vi "File_data_new.vi"(6 "Nota 3":string, 8 "Nota 2":string, 9 "Nota 01":string, 10 "Sample name":string, 11 "File name":string) -> (4 "path":path)   [LabVIEW 2011]
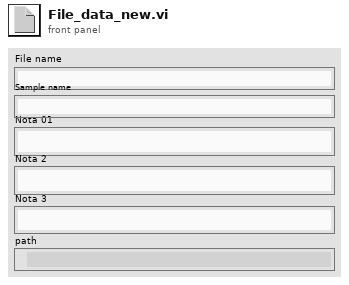
[diagram p1: front panel]
types:
  T1 = enum16{"open", "replace", "create", "open or create", "replace or create", "replace or create with confirmation"}
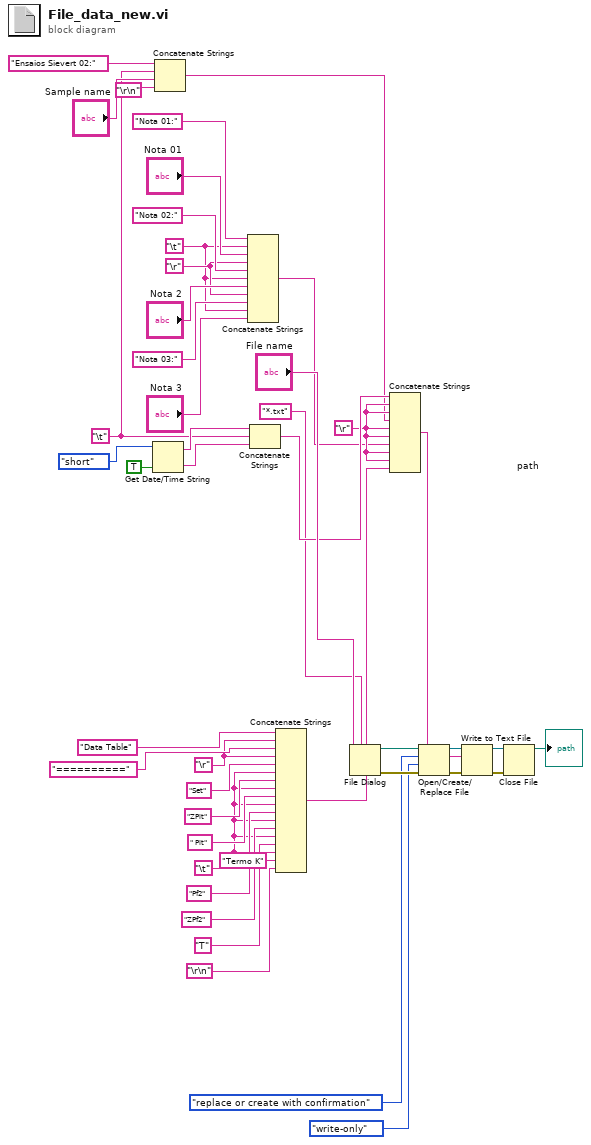
[diagram p0: block diagram]
diagram:
  w3 = "\t"
  w23 = "\r"
  w21 = "\t"
  w29 = "\r"
  w26 = "\r"
  w7 = "\t"
  n1 = Get Date/Time String(date format (0)=enum16{"short", "long", "abbreviated"}."short", want seconds? (F)=TRUE) -> (date string=w39:string, time string=w38:string)  [unwired: 1 in]
  n2 = Concatenate Strings("Ensaios Sievert 02:" ("string"), w7, "Sample name", "\r\n") -> (w5:string)
  n3 = Concatenate Strings("Nota 01:" ("Nota 4"), w21, "Nota 01", w23, "Nota 02:" ("Nota 4"), w21, "Nota 2", w23, "Nota 03:" ("Nota 4"), w21, "Nota 3") -> (w20:string)
  n4 = Concatenate Strings(w39, w7, w38) -> (w28:string)
  n5 = Concatenate Strings("Data Table" ("string"), w29, "==========" ("string"), w29, "Set" ("string"), w3, "ZPit" ("string"), w3, " Pit" ("string"), w3, "Pf2" ("string"), w3, "ZPf2" ("string"), w3, "T" ("string"), w3, "Termo K" ("string"), "\r\n") -> (w27:string)
  n6 = File Dialog(6:"*.txt" ("pattern label"), 9:"File name") -> (0:w18:errorcluster, 3:w19:path)  [unwired: 2 in, 5 out]
  n7 = Concatenate Strings(w28, w26, w26, w5, w26, w26, w20, w26, w26, w27) -> (w37:string)
  n8 = Open/Create/Replace File(file path (use dialog)=w19, error in=w18, operation (0:open)=T1."replace or create with confirmation", access (0:read/write)=enum16{"read/write", "read-only", "write-only"}."write-only") -> (refnum out=w15:refnum<file>, error out=w14:errorcluster)  [unwired: 3 out]
  n9 = Write to Text File(file (use dialog)=w15, text=w37, error in=w14) -> (refnum out=w13:refnum<file>, error out=w10:errorcluster)  [unwired: 1 in, 1 out]
  n10 = Close File(refnum=w13, error in=w10) -> (path=→"path":path)  [unwired: 1 out]
